vi "Log_beam_power.vi"(3 "Message":string, 5 "Beam Data":dbl[][](array[numeric]) format="%.2f") -> ()   [LabVIEW 2010]
uses:
  Controls/Beam_Type.ctl
panel:
  out "Server copy Location":path
  out "Log File":path
  out "Beam Type":T1 items=["Green Unshifted", "Green Shifted", "Blue Unshifted", "Blue Shifted"]
  # "X                Y                 Z                 Power"
  # "Green Unshifted\nGreen Shifted\nBlue Unshifted\nBlue Shifted"
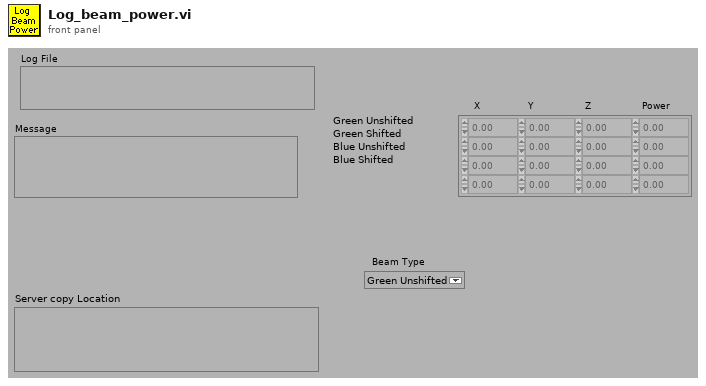
[diagram p1: front panel]
types:
  T1 = typedef "Beam_Type.ctl" = u16
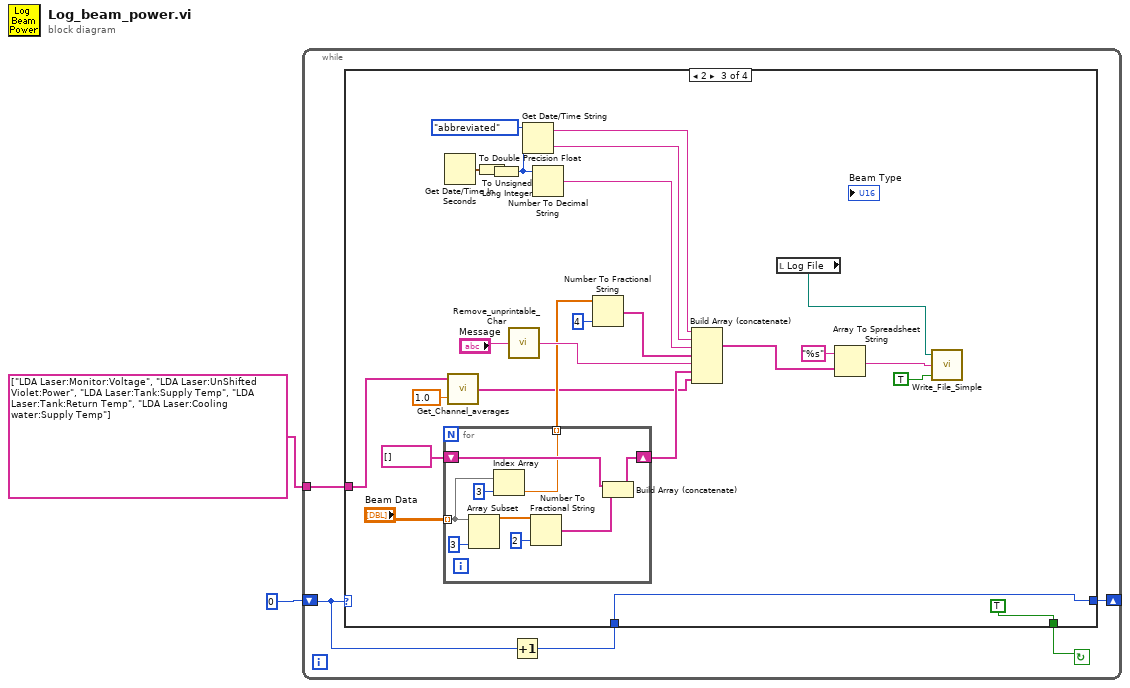
[diagram p0: block diagram]
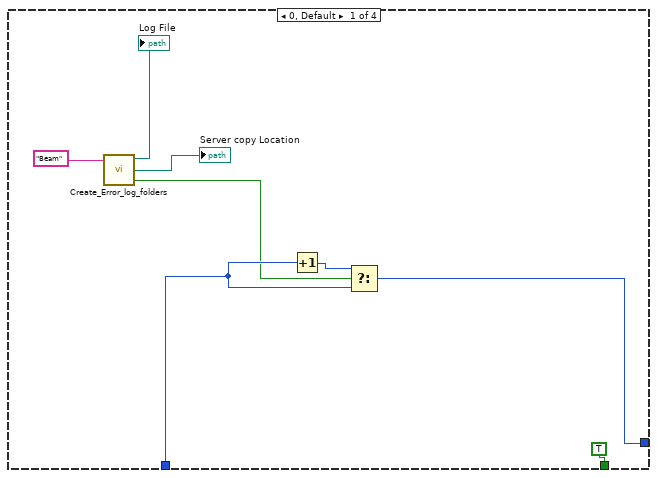
[diagram p2: hidden frame]
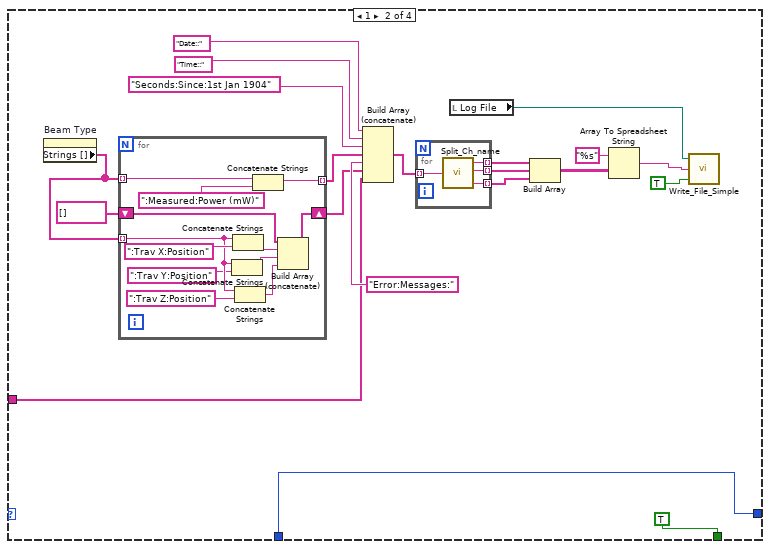
[diagram p3: hidden frame]
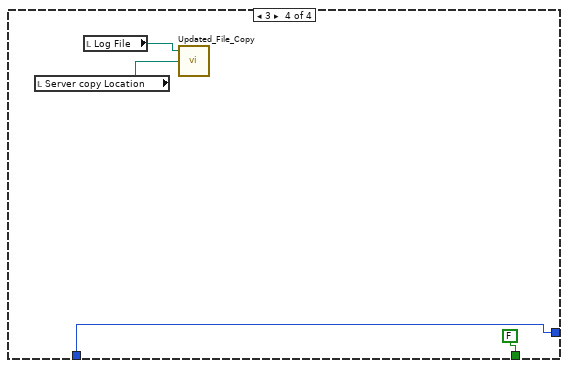
[diagram p4: hidden frame]
diagram:
  n1 = while {
    shift-left: 0 -> [w7]
    shift-right: [w4] -> _
    tunnel: string[] ["LDA Laser:Monitor:Voltage", "LDA Laser:UnShifted Violet:Power", "LDA Laser:Tank:Supply Temp", "LDA Laser:Tank:Return Temp", "LDA Laser:Cooling water:Supply Temp"] -> [w3]
    stop <- w6 continue-if-true
    n2 = Increment(x=w7) -> (x+1=w5:i32)
    n3 = case shown="2" w7 {
      tunnel: [TRUE TRUE TRUE FALSE] -> w6
      tunnel: w5 -> [w12 w23 w73 w86]
      tunnel: [w11 w23 w73 w86] -> w4
      tunnel: w3 -> [_ w16 w53 _]
      frame 0, Default {
        n4 = call "Create_Error_log_folders.vi"("Log Filename"="Beam" ("Input Element")) -> ("exists?"=w9:bool, "Server copy Location"=→"Server copy Location":path, "Local Log File"=→"Log File":path)  [unwired: 2 in]
        n5 = Increment(x=w12) -> (x+1=w14:i32)
        n6 = Select(t=w14, s=w9, f=w12) -> (s? t:f=w11:i32)
      }
      frame 1 {
        n7 = property on="Beam Type" class="Ring (strict)"() -> ("Strings []"=w21:string[])  [unwired: 2 in, 2 out]
        n8 = for {
          tunnel: w21 -> [w47] mode=indexing
          tunnel: [w45] -> w26 mode=indexing
          shift-right: [w36] -> w20
          shift-left: string[] [] -> [w40]
          tunnel: w21 -> [w43] mode=indexing
          n9 = Concatenate Strings(w43, ":Trav Y:Position") -> (w38:string)
          n10 = Concatenate Strings(w43, ":Trav X:Position") -> (w39:string)
          n11 = Concatenate Strings(w43, ":Trav Z:Position") -> (w37:string)
          n12 = Concatenate Strings(w47, ":Measured:Power (mW)") -> (w45:string)
          n13 = Build Array (concatenate)(w40, w39, w38, w37) -> (w36:string[])
        }
        n14 = Build Array (concatenate)("Date::", "Time::", "Seconds:Since:1st Jan 1904", w26, "Error:Messages:", w20, w16) -> (w29:string[])
        n15 = for {
          tunnel: w29 -> [w51] mode=indexing
          tunnel: [w50] -> w30 mode=indexing
          tunnel: [w49] -> w31 mode=indexing
          tunnel: [w48] -> w32 mode=indexing
          n16 = call "Split_Ch_name.vi"("Ch name"=w51) -> ("Top level"=w50:string, "Middle"=w49:string, "Low level"=w48:string)
        }
        n17 = local read "Log File"() -> (w17:path)
        n18 = Build Array(w30, w31, w32) -> (w27:string[][])
        n19 = Array To Spreadsheet String(array=w27, 3:"%s" ("format string")) -> (spreadsheet string=w18:string)  [unwired: 1 out]
        n20 = call "Write_File_Simple.vi"("append to file? (new file:F)"=TRUE, "character string"=w18, "file path"=w17) -> ()  [unwired: 2 out]
      }
      frame 2 {
        n21 = for {
          shift-right: [w84] -> w59
          shift-left: string[] [] -> [w85]
          tunnel: "Beam Data" -> [w78] mode=indexing
          tunnel: [w77] -> w60 mode=indexing
          n22 = Array Subset(array=w78, length=3 ("Array Length")) -> (w81:dbl[])  [unwired: 1 in]
          n23 = Index Array(array=w78, index=3 ("Index")) -> (element=w77:dbl)
          n24 = Number To Fractional String(number=w81, precision (6)=i16 2) -> (F-format string=w82:string[])  [unwired: 2 out]
          n25 = Build Array (concatenate)(w85, w82) -> (w84:string[])
        }
        n26 = Get Date/Time In Seconds() -> (seconds since 1Jan1904=w57:timestamp)
        n27 = call "Get_Channel_averages.vi"("Desired Ch Names"=w53, "Averaging time (mins)"=1.0) -> ("Values"=w52:string[])  [unwired: 1 in, 2 out]
        n28 = To Double Precision Float(number=w57) -> (double precision float=w71:dbl)
        n29 = To Unsigned Long Integer(number=w71) -> (unsigned 32bit integer=w70:u32)
        n30 = call "Remove_unprintable_Char.vi"("Input String"="Message") -> ("Output String"=w63:string)
        n31 = Get Date/Time String(date format (0)=enum16{"short", "long", "abbreviated"}."abbreviated", seconds (now)=w70) -> (date string=w69:string, time string=w68:string)  [unwired: 1 out]
        n32 = Number To Decimal String(number=w70) -> (decimal integer string=w67:string)  [unwired: 1 out]
        n33 = Number To Fractional String(number=w60, precision (6)=i16 4) -> (F-format string=w64:string[])  [unwired: 2 out]
        n34 = Build Array (concatenate)(w69, w68, w67, w64, w63, w59, w52) -> (w66:string[])
        n35 = local read "Log File"() -> (w54:path)
        n36 = Array To Spreadsheet String(array=w66, 3:"%s" ("format string")) -> (spreadsheet string=w55:string)  [unwired: 1 out]
        n37 = call "Write_File_Simple.vi"("append to file? (new file:F)"=TRUE, "character string"=w55, "file path"=w54) -> ()  [unwired: 2 out]
      }
      frame 3 {
        n38 = local read "Server copy Location"() -> (w88:path)
        n39 = local read "Log File"() -> (w89:path)
        n40 = call "Updated_File_Copy.vi"("Target Path"=w88, "Source Path"=w89) -> ()  [unwired: 2 out]
      }
    }
  }
